vi "DynamicComboBox.vi"(5 "Secondary Delay Line":string(combo)="Please Select", 6 "Primary Delay Line":string(combo)="Please Select", 7 "Strings []":string[](array[string]), 8 "error in (no error)":errorcluster) -> (0 "Secondary Delay Line Indicator":string, 1 "Primary Delay Line Indicator":string, 3 "error out":errorcluster)   [LabVIEW 2009]
panel:
  in  "stop":bool
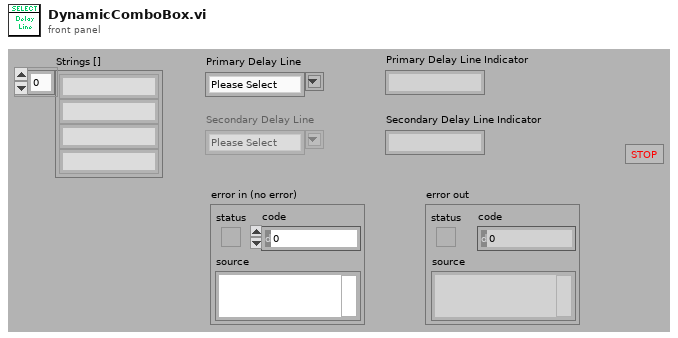
[diagram p1: front panel]
types:
  T1 = enum8{"Enabled", "Disabled", "Disabled and Grayed Out"}
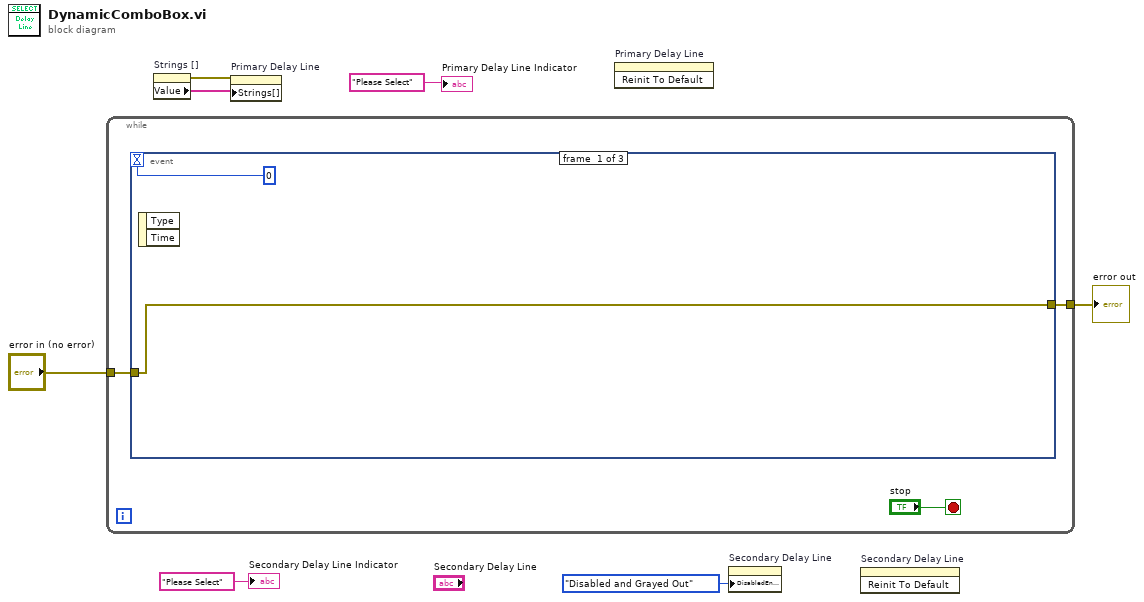
[diagram p0: block diagram]
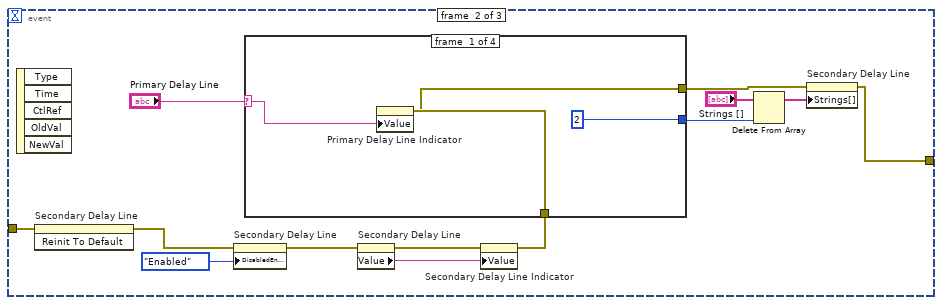
[diagram p2: hidden frame]
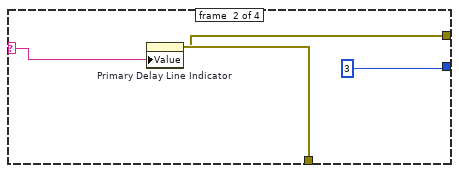
[diagram p3: hidden frame]
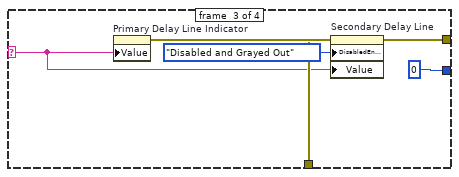
[diagram p4: hidden frame]
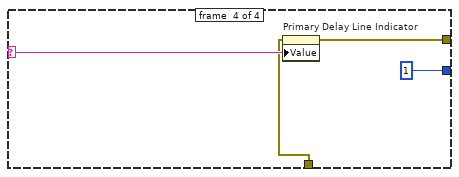
[diagram p5: hidden frame]
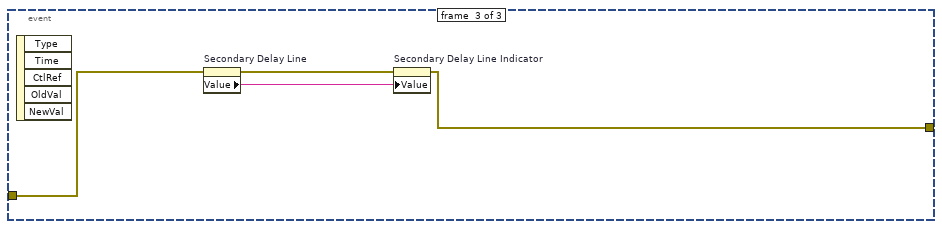
[diagram p6: hidden frame]
diagram:
  n1 = while {
    tunnel: "error in (no error)" -> [w9]
    tunnel: [w8] -> w1
    stop <- "stop" stop-if-true
    n2 = event shown="[2] \"Secondary Delay Line\": Value Change" {
      selector: _ -> [_ _ _]
      dyn-events: _ -> [_ _ _]
      timeout: 0 -> [_ _ _]
      tunnel: w9 -> [w12 w14 w44]
      tunnel: [w12 w13 w45] -> w8
      event #0 {
        n3 = event-data() -> ()  [unwired: 1 in, 2 out]
      }
      event #1 {
        n4 = event-data() -> ()  [unwired: 1 in, 5 out]
        n5 = invoke on="Secondary Delay Line" class="CmbBox" method="Reinit To Default"(error in=w14) -> (error out=w20:errorcluster)  [unwired: 2 in, 2 out]
        n6 = property on="Secondary Delay Line" class="CmbBox"(error in=w20, "DisabledEnum"=T1."Enabled" ("Disabled")) -> (error out=w16:errorcluster)  [unwired: 1 in, 1 out]
        n7 = property on="Secondary Delay Line" class="CmbBox"(error in=w16) -> (error out=w18:errorcluster, "Value"=w17:string)  [unwired: 1 in, 1 out]
        n8 = property on="Secondary Delay Line Indicator" class="Str"(error in=w18, "Value"=w17) -> (error out=w15:errorcluster)  [unwired: 1 in, 1 out]
        n9 = case shown="\"Please Select\", Default" "Primary Delay Line" {
          selector: "Primary Delay Line" -> [w27 w31 w34 w42]
          tunnel: [2 3 0 1] -> w21
          tunnel: w15 -> [w28 w32 w36 w41]
          tunnel: [w26 w30 w35 w40] -> w19
          frame #0 {
            n10 = property on="Primary Delay Line Indicator" class="Str"(error in=w28, "Value"=w27) -> (error out=w26:errorcluster)  [unwired: 1 in, 1 out]
          }
          frame #1 {
            n11 = property on="Primary Delay Line Indicator" class="Str"(error in=w32, "Value"=w31) -> (error out=w30:errorcluster)  [unwired: 1 in, 1 out]
          }
          frame #2 {
            n12 = property on="Primary Delay Line Indicator" class="Str"(error in=w36, "Value"=w34) -> (error out=w37:errorcluster)  [unwired: 1 in, 1 out]
            n13 = property on="Secondary Delay Line" class="CmbBox"(error in=w37, "DisabledEnum"=T1."Disabled and Grayed Out" ("Disabled"), "Value"=w34) -> (error out=w35:errorcluster)  [unwired: 1 in, 1 out]
          }
          frame #3 {
            n14 = property on="Primary Delay Line Indicator" class="Str"(error in=w41, "Value"=w42) -> (error out=w40:errorcluster)  [unwired: 1 in, 1 out]
          }
        }
        n15 = Delete From Array(array="Strings []", index=w21) -> (array with subset deleted=w23:string[])  [unwired: 1 in, 1 out]
        n16 = property on="Secondary Delay Line" class="CmbBox"(error in=w19, "Strings[]"=w23) -> (error out=w13:errorcluster)  [unwired: 1 in, 1 out]
      }
      event #2 {
        n17 = event-data() -> ()  [unwired: 1 in, 5 out]
        n18 = property on="Secondary Delay Line" class="CmbBox"(error in=w44) -> (error out=w46:errorcluster, "Value"=w47:string)  [unwired: 1 in, 1 out]
        n19 = property on="Secondary Delay Line Indicator" class="Str"(error in=w46, "Value"=w47) -> (error out=w45:errorcluster)  [unwired: 1 in, 1 out]
      }
    }
  }
  "error out" <- w1
  n20 = property on="Strings []" class="Arr (strict)"() -> (error out=w3:errorcluster, "Value"=w4:string[])  [unwired: 2 in, 1 out]
  n21 = property on="Primary Delay Line" class="CmbBox"(error in=w3, "Strings[]"=w4) -> ()  [unwired: 1 in, 2 out]
  n22 = invoke on="Primary Delay Line" class="CmbBox" method="Reinit To Default"() -> ()  [unwired: 3 in, 3 out]
  n23 = property on="Secondary Delay Line" class="CmbBox"("DisabledEnum"=T1."Disabled and Grayed Out" ("Disabled")) -> ()  [unwired: 2 in, 2 out]
  n24 = invoke on="Secondary Delay Line" class="CmbBox" method="Reinit To Default"() -> ()  [unwired: 3 in, 3 out]
  "Primary Delay Line Indicator" <- "Please Select"
  "Secondary Delay Line Indicator" <- "Please Select"
